vi "Merenje_3_ACC.vi"() -> ()   [LabVIEW 2016]
uses:
  <vilib>/Waveform/WDTOps.llb/WDT Index Channel DBL.vi
panel:
  in  "Enable":bool
  out "ACC 3":dynamicdata(graph)
  out "ACC 2":dynamicdata(graph)
  out "ACC 1":dynamicdata(graph)
  in  "stop (F)":bool
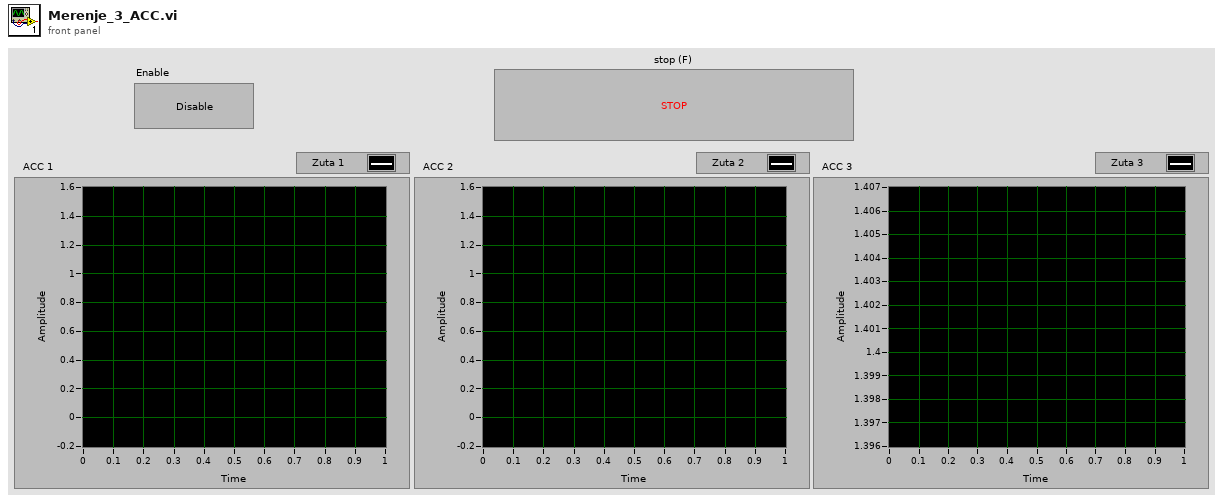
[diagram p1: front panel]
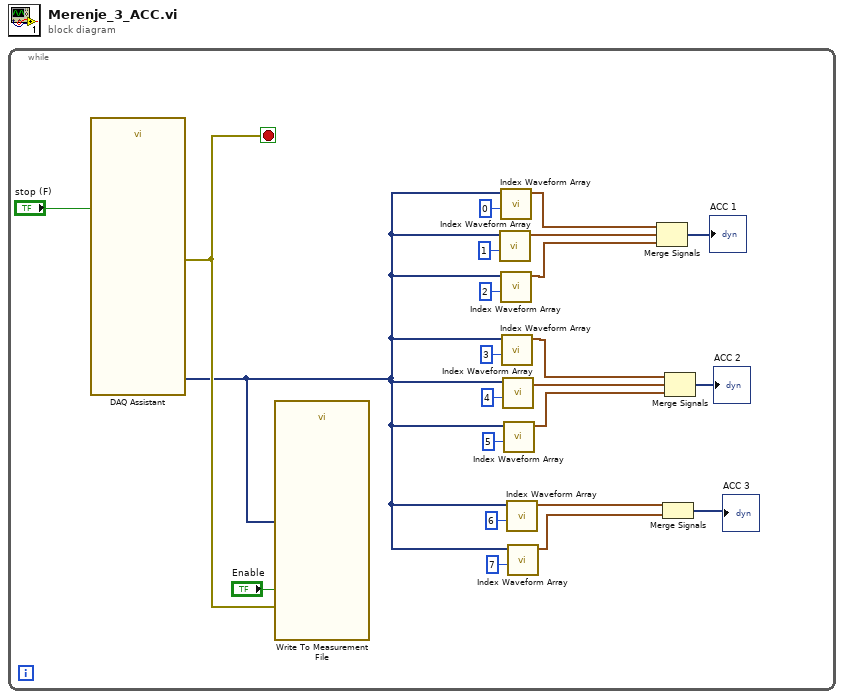
[diagram p0: block diagram]
diagram:
  n1 = while {
    stop <- w3 stop-if-true
    n2 = call "DAQ Assistant"("stop (F)"="stop (F)") -> ("data"=w2:dynamicdata, "error out"=w3:errorcluster)  [unwired: 15 in, 2 out]
    n3 = call "Write To Measurement File"("Signals"=w2, "Enable"="Enable", "error in (no error)"=w3) -> ()  [unwired: 14 in, 3 out]
    n4 = call-poly <vilib>:"Index Waveform Array.vi"("index"=1, "waveform array"=w2) -> ("waveform"=w9:waveform(dbl))  [unwired: 8 in, 1 out]
    n5 = call-poly <vilib>:"Index Waveform Array.vi"("index"=0, "waveform array"=w2) -> ("waveform"=w8:waveform(dbl))  [unwired: 8 in, 1 out]
    n6 = call-poly <vilib>:"Index Waveform Array.vi"("index"=2, "waveform array"=w2) -> ("waveform"=w7:waveform(dbl))  [unwired: 8 in, 1 out]
    n7 = call-poly <vilib>:"Index Waveform Array.vi"("index"=3, "waveform array"=w2) -> ("waveform"=w12:waveform(dbl))  [unwired: 8 in, 1 out]
    n8 = call-poly <vilib>:"Index Waveform Array.vi"("index"=4, "waveform array"=w2) -> ("waveform"=w13:waveform(dbl))  [unwired: 8 in, 1 out]
    n9 = call-poly <vilib>:"Index Waveform Array.vi"("index"=5, "waveform array"=w2) -> ("waveform"=w11:waveform(dbl))  [unwired: 8 in, 1 out]
    n10 = call-poly <vilib>:"Index Waveform Array.vi"("index"=6, "waveform array"=w2) -> ("waveform"=w6:waveform(dbl))  [unwired: 8 in, 1 out]
    n11 = call-poly <vilib>:"Index Waveform Array.vi"("index"=7, "waveform array"=w2) -> ("waveform"=w5:waveform(dbl))  [unwired: 8 in, 1 out]
    n12 = Merge Signals(w8, w9, w7) -> (→"ACC 1":dynamicdata)
    n13 = Merge Signals(w6, w5) -> (→"ACC 3":dynamicdata)
    n14 = Merge Signals(w12, w13, w11) -> (→"ACC 2":dynamicdata)
  }
